vi "Replace Error Source.vi"(7 "New Source":string, 10 "error in (no error)":errorcluster) -> (2 "error out":errorcluster)   [LabVIEW 2020, in "VolatusErrorUtilities.lvlib"]
uses:
  VolatusErrorUtilities.lvlib
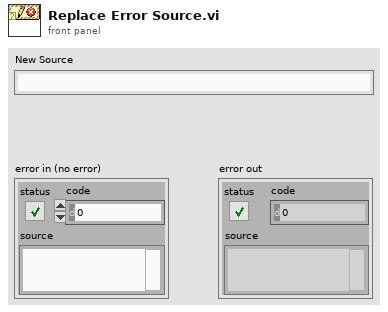
[diagram p1: front panel]
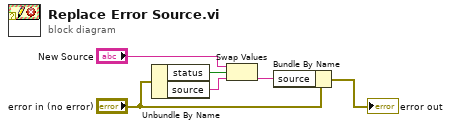
[diagram p0: block diagram]
diagram:
  n1 = Unbundle By Name("error in (no error)") -> ("status"=w3:bool, "source"=w4:string)
  n2 = Swap Values(12:"New Source", 13:w3, 14:w4) -> (3:w1:string)  [unwired: 1 out]
  n3 = Bundle By Name(cluster="error in (no error)", "source"=w1) -> (→"error out":errorcluster)
